vi "Do Core.vi"(8 "error in":errorcluster, 9 "Actor in":refnum<class "Actor.lvclass">, 11 "Reply Message":refnum<class "Get Temperature DBL Msg.lvclass">) -> (0 "error out":errorcluster, 1 "Actor out":refnum<class "Actor.lvclass">, 2 "Reply":variant)   [LabVIEW 2024, in "Thermometer Multichannel Worker.lvlib" / "Get Temperature DBL Msg.lvclass"]
doc: "<p>(<strong>Filename</strong>: <span class=\"dnl\">Actor Framework.lvlib:Reply Msg.lvclass:Do Core.vi</span>)</p>\n<p>Defines what an actor does when it receives <strong>Reply Message</strong>. This method also defines the <strong>Reply</strong> that is returned to the actor that sent <strong>Reply Message</strong>.</p>\n<p>By default, this method does nothing, and <strong>Reply</strong> is the ancestor Message class. A child class must override this method to define behavior and specify a child of the Message class to return in the <strong>Reply</strong> output.</p>"
uses:
  Get Temperature DBL Msg.lvclass
  <vilib>/ActorFramework/Actor/Actor.lvclass
  Thermometer Multichannel Worker/Thermometer Multichannel Worker.lvclass
  C:/Program Files/National Instruments/LabVIEW 2025/vi.lib/ActorFramework/Actor/Actor.lvclass
  Get Temperature DBL Msg.lvclass/Get Temperature DBL Msg.ctl
  f5df564e-eb9b-4f33-b862-635a4d0ae9c2.vi
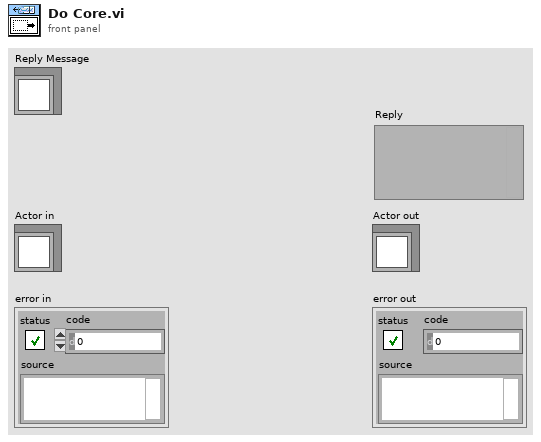
[diagram p1: front panel]
types:
  T1 = cluster{"Temperature":dbl, "Time Stamp":timestamp}
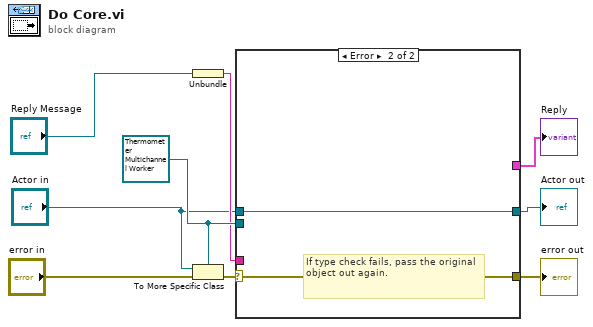
[diagram p0: block diagram]
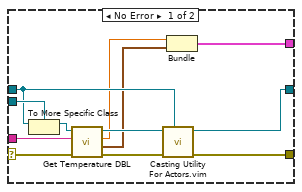
[diagram p2: hidden frame]
diagram:
  w8 = refnum<class "Thermometer Multichannel Worker.lvclass"> refnum ("Actor in")
  n1 = Unbundle("Reply Message") -> (w7:string)
  n2 = To More Specific Class(target class=w8, reference="Actor in", error in="error in") -> (error out=w9:errorcluster)  [unwired: 1 out]
  n3 = case shown="Error" w9 {
    selector: w9 -> [w21 w23]
    tunnel: [w15 w23] -> w6
    tunnel: [w16 w22] -> w1
    tunnel: "Actor in" -> [w18 w22]
    tunnel: w8 -> [w19 _]
    tunnel: w7 -> [w13 _]
    tunnel: [w10 _] -> w2
    frame No Error {
      n4 = To More Specific Class(target class=w19, reference=w18) -> (specific class reference=w20:refnum<class "Thermometer Multichannel Worker.lvclass">)  [unwired: 1 in, 1 out]
      n5 = call-dynamic "Get Temperature DBL.vi"("error in"=w21, "Source"=w13, "Thermometer Multichannel Worker in"=w20) -> ("error out"=w14:errorcluster, "Time Stamp"=w11:timestamp, "Temperature"=w12:dbl, "Thermometer Multichannel Worker out"=w17:refnum<class "Thermometer Multichannel Worker.lvclass">)  [unwired: 5 in]
      n6 = call "Casting Utility For Actors.vim"("type"=w18, "error in (no error)"=w14, "Actor in"=w17) -> ("error out"=w15:errorcluster, "Actor out"=w16:refnum<class "Actor.lvclass">)  [unwired: 7 in]
      n7 = Bundle("Temperature"=w12, "Time Stamp"=w11) -> (w10:T1)  [unwired: 1 in]
    }
    frame Error {
      # "If type check fails, pass the original object out again."
    }
  }
  "error out" <- w6
  "Actor out" <- w1
  "Reply" <- w2
